vi "Raycaster_DrawColumnTextured.vi"(4 "Sub Buffer":u8, 6 "column":u32, 8 "Buffer In":u8[](array[numeric]), 9 "Location Info":T2, 10 "Column Calcs":T1, 11 "DDA Calculation In":T4) -> (0 "Buffer Out":u8[](array[numeric]))   [LabVIEW 2020]
uses:
  Controls/Raycaster_DDACalcs.ctl
  Controls/Raycaster_WallColumnAxis.ctl
  Controls/Player_LocationInfo.ctl
  Controls/Player_LocationInfoAxis.ctl
  Controls/Raycaster_ScreenCalcs.ctl
  Texture_GetTextures.vi
  <vilib>/Utility/file.llb/Application Directory.vi
  <vilib>/picture/bmp.llb/Read BMP File.vi
  <vilib>/rvi/DataTransferAndStorage/Container/XNode/niFpgaContainer.xnode
  <vilib>/rvi/DataTransferAndStorage/Register/Emulation/niFpgaRegisterEmulation.vi
  <vilib>/Platform/TimedLoop/XDataNode/XDataNode.xnode
  <vilib>/Platform/TimedLoop/XDataNode/nitl_modes.ctl
  <vilib>/Platform/TimedLoop/XDataNode/XDNodeRunTimeDep.lvlib
  <vilib>/Platform/TimedLoop/XDataNode/wakeup.ctl
  <vilib>/Platform/TimedLoop/XDataNode/timing_clust.ctl
  <vilib>/rvi/Memory/Memory_Emulation/nirvimemoryFastEmulation.vi
  <vilib>/rvi/Memory/Memory_Emulation/nirvimemoryEmulation.vi
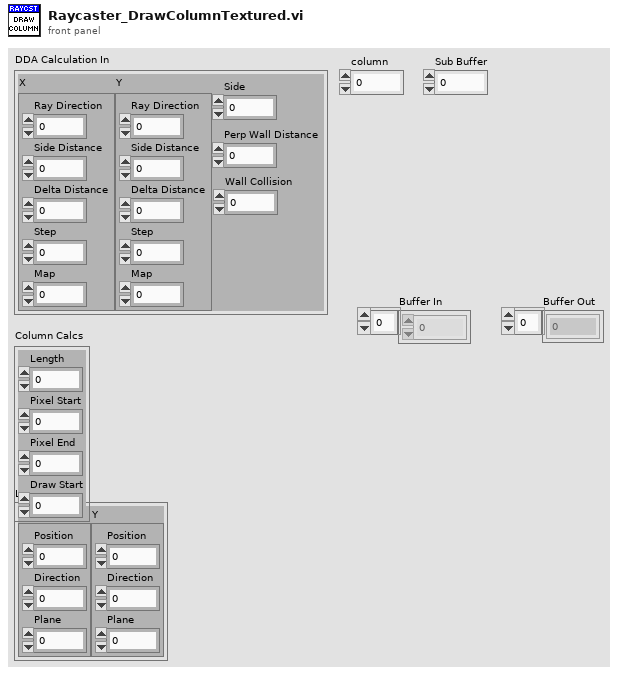
[diagram p1: front panel]
types:
  T1 = typedef "Raycaster_ScreenCalcs.ctl" = cluster{"Length":i16, "Pixel Start":i16, "Pixel End":i16, "Draw Start":i16}
  T2 = typedef "Player_LocationInfo.ctl" = cluster{"X":T3, "Y":T3}
  T3 = typedef "Player_LocationInfoAxis.ctl" = cluster{"Position":fxp<+/-,32,16>, "Direction":fxp<+/-,32,16>, "Plane":fxp<+/-,32,16>}
  T4 = typedef "Raycaster_DDACalcs.ctl" = cluster{"X":T5, "Y":T5, "Side":u8, "Perp Wall Distance":fxp<+/-,32,16>, "Wall Collision":u8}
  T5 = typedef "Raycaster_WallColumnAxis.ctl" = cluster{"Ray Direction":fxp<+/-,32,16>, "Side Distance":fxp<+/-,32,16>, "Delta Distance":fxp<+/-,32,16>, "Step":i16, "Map":i16}
  T6 = typedef "XDNodeRunTimeDep.lvlib/timing_clust.ctl" = cluster{"Expected End [f-1]":u64, "Actual End [f-1]":u64, "Finished Late? [f-1]":bool, "Expected End [i-1]":u64, "Actual End [i-1]":u64, "Finished Late? [i-1]":bool, "Expected Start [i]":u64, "Actual Start [i]":u64, "Expected Start [f]":u64, "Actual Start [f]":u64, "Source Name":string, "Structure Name":string, "Period":i64, "Deadline":i64, "Offset":i64, "Start":i64, "Priority":i32, "Timeout":i32, "Mode":T7, "Wakeup Reason":T8, "Error":errorcluster, "Source Type":string, "Secondary Source Type":string, "Global End Time":u64, "Global Start Time":u64, "Frame Duration":u64, "Iteration Duration":u64, "Assigned CPU":i32, "I/O Scan Engine Mode":u32}
  T7 = typedef "XDNodeRunTimeDep.lvlib/nitl_modes.ctl" = enum32{"No Change", "Process missed periods, maintain original phase", "Discard missed periods, maintain original phase", "Process missed periods, ignore original phase", "Discard missed periods, ignore original phase"}
  T8 = typedef "XDNodeRunTimeDep.lvlib/wakeup.ctl" = enum32{"Normal", "Aborted", "Asynchronous wakeup", "Timing source error", "Timed loop error", "Timeout"}
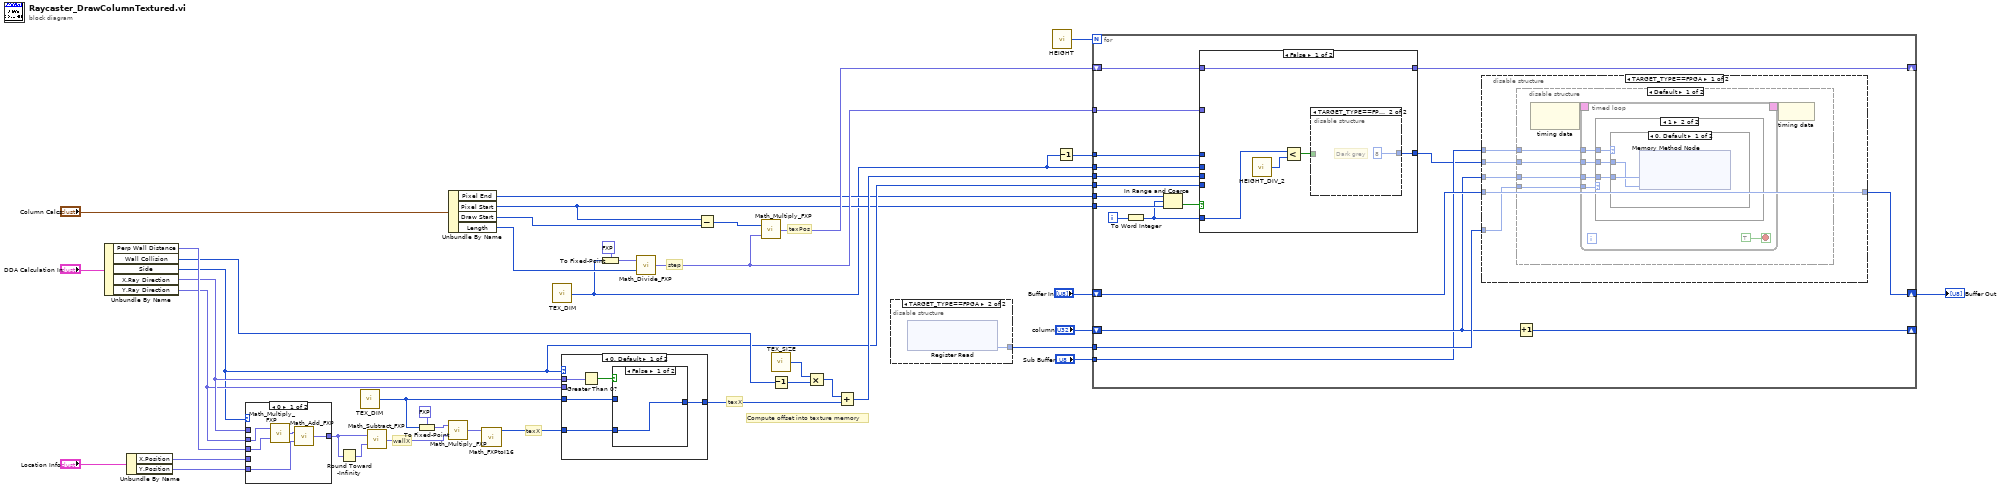
[diagram p0: block diagram]
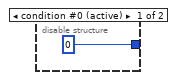
[diagram p2: hidden frame]
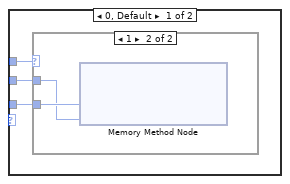
[diagram p3: hidden frame]
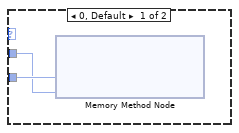
[diagram p4: hidden frame]
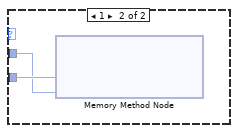
[diagram p5: hidden frame]
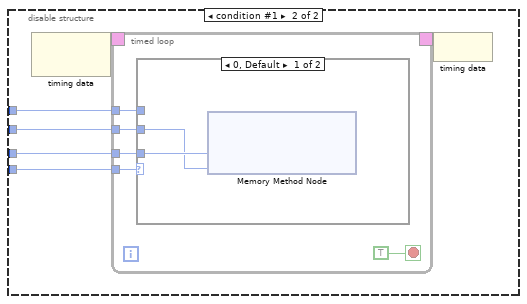
[diagram p6: hidden frame]
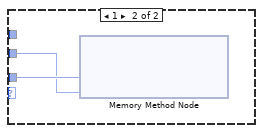
[diagram p7: hidden frame]
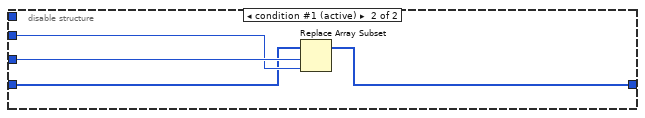
[diagram p8: hidden frame]
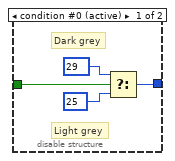
[diagram p9: hidden frame]
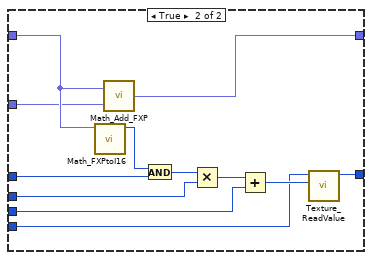
[diagram p10: hidden frame]
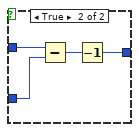
[diagram p11: hidden frame]
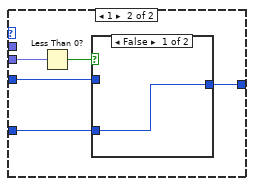
[diagram p12: hidden frame]
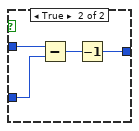
[diagram p13: hidden frame]
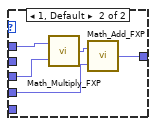
[diagram p14: hidden frame]
diagram:
  # "Compute offset into texture memory"
  # "texPos"
  # "step"
  # "texX"
  # "texX"
  # "wallX"
  n1 = Unbundle By Name("DDA Calculation In") -> ("Perp Wall Distance"=w38:fxp<+/-,32,16>, "Wall Collision"=w22:u8, "Side"=w10:u8, "X.Ray Direction"=w34:fxp<+/-,32,16>, "Y.Ray Direction"=w33:fxp<+/-,32,16>)
  n2 = Unbundle By Name("Location Info") -> ("X.Position"=w40:fxp<+/-,32,16>, "Y.Position"=w39:fxp<+/-,32,16>)
  n3 = case shown="0" w10 {
    tunnel: w34 -> [_ w49]
    tunnel: w33 -> [w42 _]
    tunnel: w40 -> [_ w46]
    tunnel: w39 -> [w41 _]
    tunnel: w38 -> [w45 w50]
    tunnel: [w43 w47] -> w37
    frame 0 {
      n4 = call "Math_Multiply_FXP.vi"("y"=w45, "x"=w42) -> ("x*y"=w44:fxp<+/-,32,16>)
      n5 = call "Math_Add_FXP.vi"("y"=w41, "x"=w44) -> ("x*y"=w43:fxp<+/-,32,16>)
    }
    frame 1, Default {
      n6 = call "Math_Multiply_FXP.vi"("y"=w50, "x"=w49) -> ("x*y"=w48:fxp<+/-,32,16>)
      n7 = call "Math_Add_FXP.vi"("y"=w46, "x"=w48) -> ("x*y"=w47:fxp<+/-,32,16>)
    }
  }
  n8 = Round Toward -Infinity(1:w37) -> (0:w36:fxp<+/-,16,16>)
  n9 = call "TEX_DIM.vi"() -> ("TEX_DIM"=w30:i16)
  n10 = call "Math_Subtract_FXP.vi"("y"=w36, "x"=w37) -> ("x*y"=w35:fxp<+/-,32,16>)
  n11 = To Fixed-Point(fixed-point type=fxp<+/-,32,16> 0.0, number=w30) -> (fixed-point=w32:fxp<+/-,32,16>)
  n12 = Unbundle By Name("Column Calcs") -> ("Pixel End"=w6:i16, "Pixel Start"=w5:i16, "Draw Start"=w2:i16, "Length"=w27:i16)
  n13 = call "Math_Multiply_FXP.vi"("y"=w35, "x"=w32) -> ("x*y"=w26:fxp<+/-,32,16>)
  n14 = call "Math_FXPtoI16.vi"("FXP"=w26) -> ("I16"=w25:i16)  [unwired: 10 in]
  n15 = call "TEX_DIM.vi"() -> ("TEX_DIM"=w4:i16)
  n16 = case shown="0, Default" w10 {
    tunnel: w25 -> [w53 w64]
    tunnel: w34 -> [w55 _]
    tunnel: w33 -> [_ w61]
    tunnel: w30 -> [w52 w63]
    tunnel: [w51 w62] -> w20
    frame 0, Default {
      n17 = Greater Than 0?(x=w55) -> (x > 0?=w54:bool)
      n18 = case shown="False" w54 {
        tunnel: w53 -> [w56 w59]
        tunnel: w52 -> [_ w60]
        tunnel: [w56 w57] -> w51
        frame False {
        }
        frame True {
          n19 = Subtract(x=w60, y=w59) -> (x-y=w58:i16)
          n20 = Decrement(x=w58) -> (x-1=w57:i16)
        }
      }
    }
    frame 1 {
      n21 = Less Than 0?(x=w61) -> (x < 0?=w65:bool)
      n22 = case shown="False" w65 {
        tunnel: w64 -> [w66 w69]
        tunnel: w63 -> [_ w70]
        tunnel: [w66 w67] -> w62
        frame False {
        }
        frame True {
          n23 = Subtract(x=w70, y=w69) -> (x-y=w68:i16)
          n24 = Decrement(x=w68) -> (x-1=w67:i16)
        }
      }
    }
  }
  n25 = To Fixed-Point(fixed-point type=fxp<+/-,32,16> 0.0, number=w4) -> (fixed-point=w28:fxp<+/-,32,16>)
  n26 = call "Math_Divide_FXP.vi"("y"=w27, "x"=w28) -> ("x*y"=w12:fxp<+/-,32,16>)
  n27 = Subtract(x=w5, y=w2) -> (x-y=w1:i16)
  n28 = call "Math_Multiply_FXP.vi"("y"=w12, "x"=w1) -> ("x*y"=w13:fxp<+/-,32,16>)
  n29 = call "TEX_SIZE.vi"() -> ("TEX_SIZE"=w23:u32)
  n30 = Decrement(x=w22) -> (x-1=w24:u8)
  n31 = Multiply(x=w23, y=w24) -> (x*y=w21:u32)
  n32 = Add(x=w21, y=w20) -> (x+y=w11:u32)
  n33 = disable-structure "Conditional Disable Structure" shown="TARGET_TYPE==FPGA" {
    disable-tunnel: [u8 0 ("Data") w72] -> w14
    frame condition #0 (active) {
    }
    frame condition #1 {
      n34 = xnode ("Register Read")() -> ("Data"=w72:u8)  [unwired: 1 in, 1 out]
    }
  }
  n35 = call "HEIGHT.vi"() -> ("HEIGHT"=w16:i16)
  n36 = Decrement(x=w4) -> (x-1=w3:i16)
  n37 = for {
    N: w16 -> [_]
    tunnel: w5 -> [w90]
    tunnel: w6 -> [w89]
    tunnel: w14 -> [w77]
    shift-right: [w87] -> _
    shift-left: "column" -> [w76]
    shift-right: [w86] -> _
    shift-left: w13 -> [w85]
    tunnel: w12 -> [w84]
    tunnel: w3 -> [w83]
    tunnel: w4 -> [w82]
    tunnel: w11 -> [w81]
    tunnel: w10 -> [w80]
    shift-right: [w78] -> w8
    shift-left: "Buffer In" -> [w79]
    tunnel: "Sub Buffer" -> [w75]
    i -> [w91]
    n38 = To Word Integer(number=w91) -> (16bit integer=w88:i16)
    n39 = In Range and Coerce(upper limit=w89, x=w88, lower limit=w90) -> (In Range?=w73:bool)  [unwired: 1 out]
    n40 = case shown="False" w73 {
      tunnel: w88 -> [w151 _]
      tunnel: [w150 w166] -> w74
      tunnel: [w149 w165] -> w86
      tunnel: w85 -> [w149 w164]
      tunnel: w84 -> [_ w163]
      tunnel: w83 -> [_ w162]
      tunnel: w82 -> [_ w161]
      tunnel: w81 -> [_ w160]
      tunnel: w80 -> [_ w159]
      frame False {
        n41 = call "HEIGHT_DIV_2.vi"() -> ("HEIGHT_DIV_2"=w153:i16)
        n42 = Less?(x=w151, y=w153) -> (x < y?=w152:bool)
        n43 = disable-structure shown="TARGET_TYPE==FPGA" {
          disable-tunnel: w152 -> [w155 _]
          disable-tunnel: [w154 u8 8] -> w150
          frame condition #0 (active) {
            # "Dark grey"
            # "Light grey"
            n44 = Select(t=u8 29, s=w155, f=u8 25) -> (s? t:f=w154:u8)
          }
          frame condition #1 {
            # "Dark grey"
          }
        }
      }
      frame True {
        n45 = call "Math_FXPtoI16.vi"("FXP"=w164) -> ("I16"=w168:i16)  [unwired: 10 in]
        n46 = call "Math_Add_FXP.vi"("y"=w163, "x"=w164) -> ("x*y"=w165:fxp<+/-,32,16>)
        n47 = And(x=w168, y=w162) -> (x .and. y?=w170:i16)
        n48 = Multiply(x=w170, y=w161) -> (x*y=w169:i16)
        n49 = Add(x=w169, y=w160) -> (x+y=w167:u32)
        n50 = call "Texture_ReadValue.vi"("Address"=w167, "Texture Bank"=w159) -> ("Value"=w166:u8)  [unwired: 9 in]
      }
    }
    n51 = disable-structure shown="TARGET_TYPE==FPGA" {
      disable-tunnel: w75 -> [w93 _]
      disable-tunnel: w76 -> [w95 w148]
      disable-tunnel: w74 -> [w96 w147]
      disable-tunnel: w79 -> [w94 w146]
      disable-tunnel: [w94 w145] -> w78
      disable-tunnel: w77 -> [w92 _]
      frame condition #0 {
        n52 = disable-structure shown="Default" {
          disable-tunnel: w96 -> [w100 w129]
          disable-tunnel: w95 -> [w99 w128]
          disable-tunnel: w93 -> [w98 w127]
          disable-tunnel: w92 -> [w97 w126]
          frame condition #0 (active) {
            n53 = node-c288() -> (w102:T6)  [unwired: 1 in]
            n54 = timed-loop {
              timing: w102 -> [_]
              timing-out: [_] -> w101
              tunnel: w97 -> [w106]
              tunnel: w99 -> [w105]
              tunnel: w100 -> [w104]
              tunnel: w98 -> [w103]
              stop <- TRUE stop-if-true
              n55 = case shown="1" w106 {
                tunnel: w105 -> [w110 w117]
                tunnel: w104 -> [w109 w116]
                tunnel: w103 -> [w108 w115]
                frame 0, Default {
                  n56 = case shown="1" w108 {
                    tunnel: w110 -> [w112 w114]
                    tunnel: w109 -> [w111 w113]
                    frame 0, Default {
                      n57 = xnode ("Memory Method Node")("Address"=w112, "Data"=w111) -> ()  [unwired: 1 in, 1 out]
                    }
                    frame 1 {
                      n58 = xnode ("Memory Method Node")("Address"=w114, "Data"=w113) -> ()  [unwired: 1 in, 1 out]
                    }
                  }
                }
                frame 1 {
                  n59 = case shown="0, Default" w115 {
                    tunnel: w117 -> [w119 w121]
                    tunnel: w116 -> [w118 w120]
                    frame 0, Default {
                      n60 = xnode ("Memory Method Node")("Address"=w119, "Data"=w118) -> ()  [unwired: 1 in, 1 out]
                    }
                    frame 1 {
                      n61 = xnode ("Memory Method Node")("Address"=w121, "Data"=w120) -> ()  [unwired: 1 in, 1 out]
                    }
                  }
                }
              }
            }
            n62 = node-c288(w101) -> ()
          }
          frame condition #1 {
            n63 = node-c288() -> (w131:T6)  [unwired: 1 in]
            n64 = timed-loop {
              timing: w131 -> [_]
              timing-out: [_] -> w130
              tunnel: w126 -> [w135]
              tunnel: w128 -> [w134]
              tunnel: w129 -> [w133]
              tunnel: w127 -> [w132]
              stop <- TRUE stop-if-true
              n65 = case shown="0, Default" w135 {
                tunnel: w134 -> [w138 w140]
                tunnel: w133 -> [w137 w139]
                tunnel: w132 -> [_ _]
                frame 0, Default {
                  n66 = xnode ("Memory Method Node")("Address"=w138, "Data"=w137) -> ()  [unwired: 1 in, 1 out]
                }
                frame 1 {
                  n67 = xnode ("Memory Method Node")("Address"=w140, "Data"=w139) -> ()  [unwired: 1 in, 1 out]
                }
              }
            }
            n68 = node-c288(w130) -> ()
          }
        }
      }
      frame condition #1 (active) {
        n69 = Replace Array Subset(array=w146, new element=w147, index=w148) -> (w145:u8[])
      }
    }
    n70 = Increment(x=w76) -> (x+1=w87:u32)
  }
  "Buffer Out" <- w8
